vi "Kinect Demo.vi"() -> ()   [LabVIEW 2011]
panel:
  out "Video Image Pixels (U32)":u32[][](array[numeric])
  out "Depth Image Pixels (U16)":u16[][](array[numeric])
  out "Video":T1(plugin-control)
  in  "stop":bool
  out "Depth":T1(plugin-control)
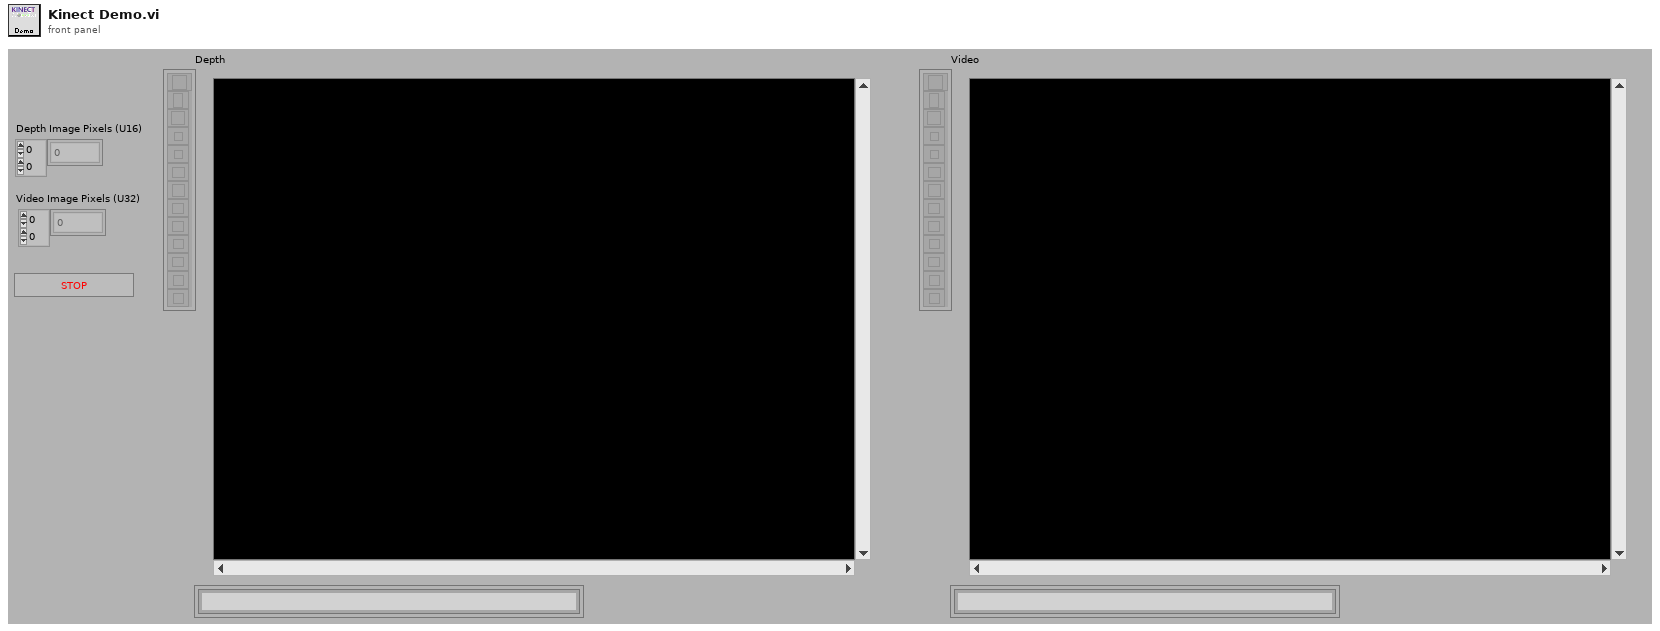
[diagram p1: front panel]
types:
  T1 = typedef "IMAQ Image.ctl" = refnum<image>
  T2 = cluster{cluster{"queue out":refnum<queue>, "queue out":refnum<queue>}, cluster{"new reference":refnum<k24>, "DepthStream":refnum<k24>, "VideoStream":refnum<k24>, "Event Callback":refnum<k27>, "Event Callback":refnum<k27>}}
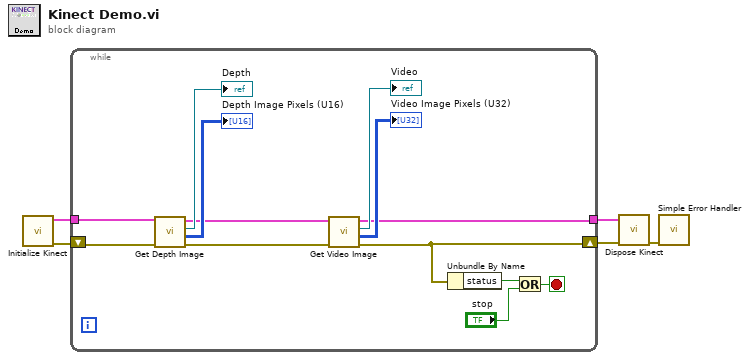
[diagram p0: block diagram]
diagram:
  n1 = call "Initialize Kinect.vi"() -> ("error out"=w5:errorcluster, "Reference Out"=w3:T2)  [unwired: 10 in]
  n2 = while {
    shift-right: [w8] -> w1
    shift-left: w5 -> [w6]
    tunnel: w3 -> [w11]
    tunnel: [w9] -> w2
    stop <- w16 stop-if-true
    n3 = call "Get Depth Image.vi"("error in (no error)"=w6, "Reference In"=w11) -> ("error out"=w7:errorcluster, "Depth Image Pixels (U16)"=→"Depth Image Pixels (U16)":u16[][], "Depth Image"=→"Depth":T1, "Reference Out"=w10:T2)  [unwired: 6 in]
    n4 = call "Get Video Image.vi"("error in (no error)"=w7, "Reference In"=w10) -> ("error out"=w8:errorcluster, "Video Image Pixels (U32)"=→"Video Image Pixels (U32)":u32[][], "Video Image"=→"Video":T1, "Reference Out"=w9:T2)  [unwired: 6 in]
    n5 = Unbundle By Name(w8) -> ("status"=w18:bool)
    n6 = Or(x=w18, y="stop") -> (x .or. y?=w16:bool)
  }
  n7 = call "Dispose Kinect.vi"("error in (no error)"=w1, "Reference In"=w2) -> ("error out"=w4:errorcluster)  [unwired: 5 in]
  n8 = call <vilib>:"Simple Error Handler.vi"("error in (no error)"=w4) -> ()  [unwired: 4 in, 5 out]
